vi "15_2c.vi"() -> ()   [LabVIEW 2020]
panel:
  in  "Turn":i32=30000000
  out "element":i32=18929178
  in  "Input":string="2,1,10,11,0,6"
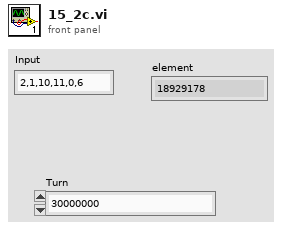
[diagram p1: front panel]
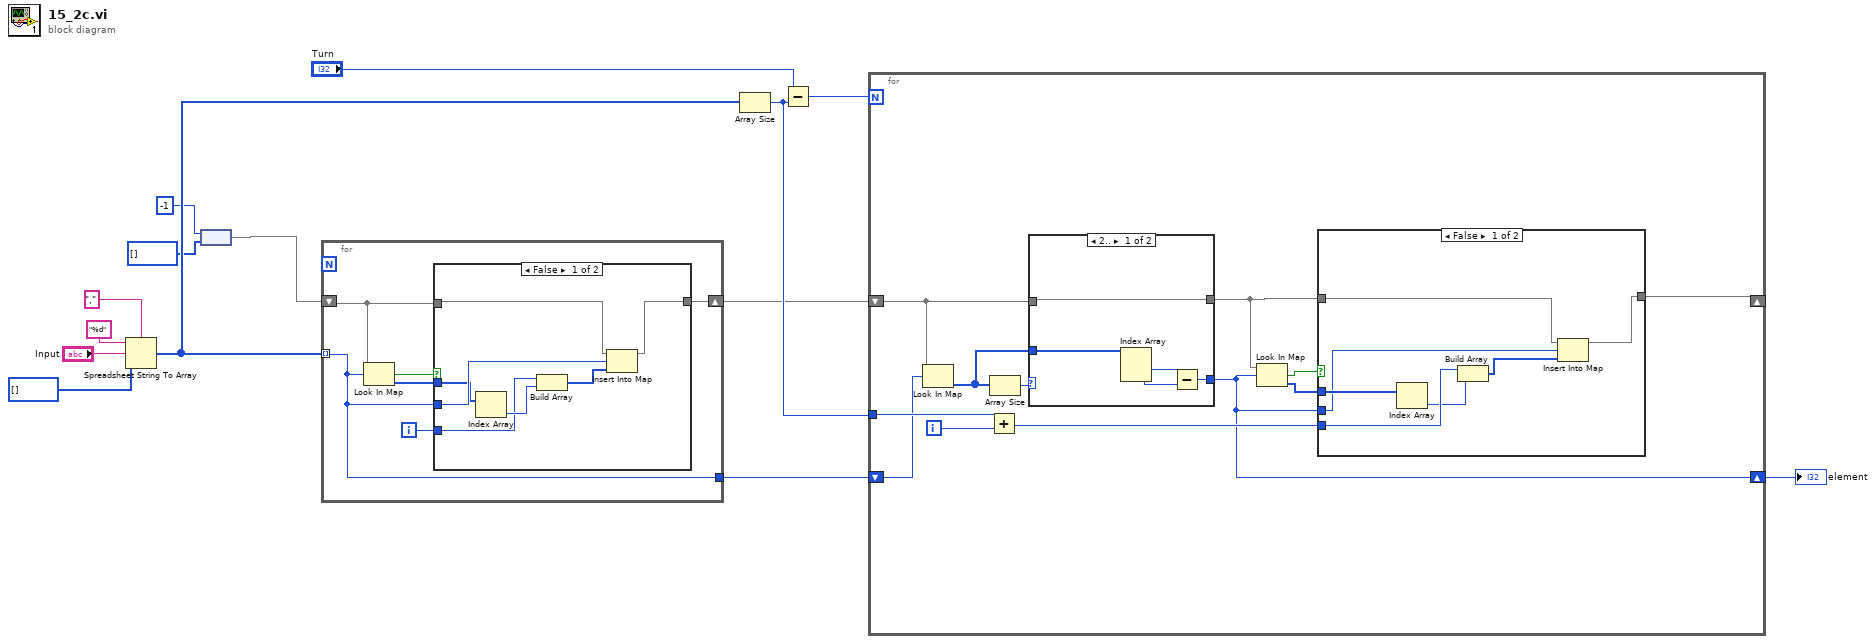
[diagram p0: block diagram]
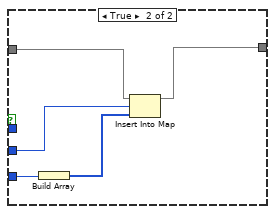
[diagram p2: hidden frame]
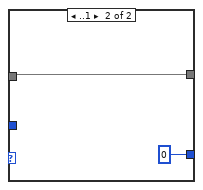
[diagram p3: hidden frame]
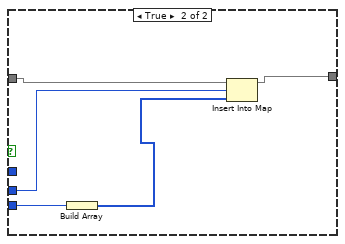
[diagram p4: hidden frame]
diagram:
  n1 = Spreadsheet String To Array(delimiter (Tab)=",", format string="%d", spreadsheet string="Input", array type (2D Dbl)=i32[] []) -> (array=w8:i32[])
  n2 = node(-1, i32[] []) -> (w2:map{i32, i32[]})
  n3 = for {
    tunnel: w8 -> [w17] mode=indexing
    shift-right: [w19] -> w1
    shift-left: w2 -> [w20]
    tunnel: [w17] -> w7
    i -> [w18]
    n4 = Look In Map(map=w20, key=w17) -> (key not found?=w16:bool, value=w15:i32[])  [unwired: 1 in]
    n5 = case shown="False" w16 {
      tunnel: w20 -> [w22 w32]
      tunnel: [w21 w28] -> w19
      tunnel: w18 -> [w24 w29]
      tunnel: w17 -> [w27 w30]
      tunnel: w15 -> [w25 _]
      frame False {
        n6 = Index Array(array=w25) -> (element=w26:i32)  [unwired: 1 in]
        n7 = Build Array(w24, w26) -> (w23:i32[])
        n8 = Insert Into Map(map in=w22, key=w27, value=w23) -> (map out=w21:map{i32, i32[]})  [unwired: 2 out]
      }
      frame True {
        n9 = Build Array(w29) -> (w31:i32[])
        n10 = Insert Into Map(map in=w32, key=w30, value=w31) -> (map out=w28:map{i32, i32[]})  [unwired: 2 out]
      }
    }
  }
  n11 = Array Size(array=w8) -> (size(s)=w5:i32)
  n12 = Subtract(x="Turn", y=w5) -> (x-y=w9:i32)
  n13 = for {
    N: w9 -> [_]
    shift-right: [w40] -> _
    shift-left: w1 -> [w44]
    shift-right: [w36] -> w6
    shift-left: w7 -> [w38]
    tunnel: w5 -> [w42]
    i -> [w43]
    n14 = Look In Map(map=w44, key=w38) -> (value=w37:i32[])  [unwired: 1 in, 1 out]
    n15 = Add(x=w42, y=w43) -> (x+y=w39:i32)
    n16 = Array Size(array=w37) -> (size(s)=w41:i32)
    n17 = case shown="2.." w41 {
      tunnel: w44 -> [w48 w50]
      tunnel: [w48 w50] -> w35
      tunnel: w37 -> [w47 _]
      tunnel: [w49 0] -> w36
      frame 2.. {
        n18 = Index Array(array=w47) -> (element #1=w46:i32, element #2=w45:i32)  [unwired: 2 in]
        n19 = Subtract(x=w46, y=w45) -> (x-y=w49:i32)
      }
      frame ..1 {
      }
    }
    n20 = Look In Map(map=w35, key=w36) -> (key not found?=w34:bool, value=w33:i32[])  [unwired: 1 in]
    n21 = case shown="False" w34 {
      tunnel: [w53 w60] -> w40
      tunnel: w35 -> [w54 w61]
      tunnel: w39 -> [w58 w63]
      tunnel: w36 -> [w55 w62]
      tunnel: w33 -> [w56 _]
      frame False {
        n22 = Index Array(array=w56) -> (element=w57:i32)  [unwired: 1 in]
        n23 = Build Array(w58, w57) -> (w52:i32[])
        n24 = Insert Into Map(map in=w54, key=w55, value=w52) -> (map out=w53:map{i32, i32[]})  [unwired: 2 out]
      }
      frame True {
        n25 = Build Array(w63) -> (w59:i32[])
        n26 = Insert Into Map(map in=w61, key=w62, value=w59) -> (map out=w60:map{i32, i32[]})  [unwired: 2 out]
      }
    }
  }
  "element" <- w6
